vi "ast_reql_response_get.vi"(8 "error in (no error)":errorcluster, 11 "reql_id in":u32 format="%08x") -> (0 "error out":errorcluster, 2 "response":string, 3 "reql_id out":u32 format="%08x")   [LabVIEW 2017]
uses:
  ast_reql_cache_action.ctl
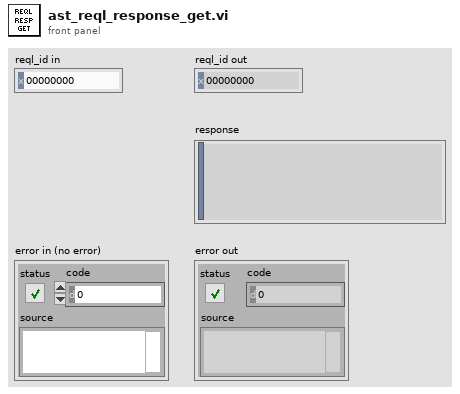
[diagram p1: front panel]
types:
  T1 = typedef "ast_reql_cache_action.ctl" = enum8{"null", "new", "get_query", "get_response", "set_query", "set_response", "delete"}
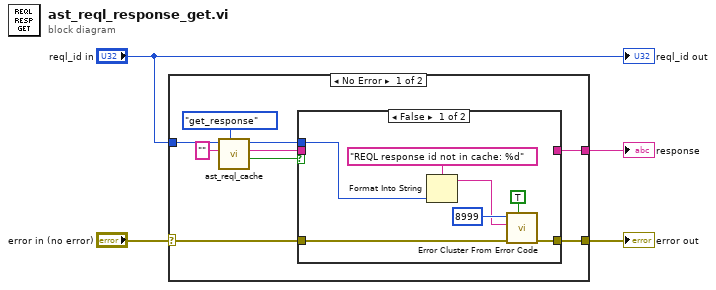
[diagram p0: block diagram]
diagram:
  n1 = case shown="No Error" "error in (no error)" {
    selector: "error in (no error)" -> [w6 w23]
    tunnel: "reql_id in" -> [w5 _]
    tunnel: [w9 _] -> w4
    tunnel: [w7 w23] -> w3
    frame No Error {
      n2 = call "ast_reql_cache.vi"("action"=ast_reql_cache_action."get_response", "query in"="" ("cmd in"), "reql_id in"=w5) -> ("exists?"=w10:bool, "query out"=w8:string, "reql_id out"=w11:u32)  [unwired: 6 in]
      n3 = case shown="False" w10 {
        tunnel: w11 -> [w14 _]
        tunnel: [_ w21] -> w9
        tunnel: w8 -> [_ w21]
        tunnel: [w19 w22] -> w7
        tunnel: w6 -> [w20 w22]
        frame False {
          n4 = Format Into String(format string="REQL response id not in cache: %d" ("error message (\"\")"), w14) -> (resulting string=w15:string)  [unwired: 2 in, 1 out]
          n5 = call <vilib>:"Error Cluster From Error Code.vi"("show call chain? (False)"=TRUE, "error in (no error)"=w20, "error message (\"\")"=w15, "error code (0)"=8999) -> ("error out"=w19:errorcluster)  [unwired: 5 in]
        }
        frame True {
        }
      }
    }
    frame Error {
    }
  }
  "response" <- w4
  "error out" <- w3
  "reql_id out" <- "reql_id in"
